vi "MouseMove.vi"(8 "Coords":T1, 9 "ActTool":i32, 10 "StartPoints":cluster{i16, i16}[](array[cluster]), 11 "reference":refnum<vi>) -> ()   [LabVIEW 2015, in "MyGraph.xctl"]
uses:
  MyGraph.xctl
  <vilib>/Utility/miscctls.llb/LVPoint32TypeDef.ctl
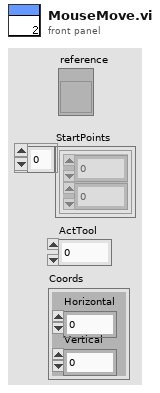
[diagram p1: front panel]
types:
  T1 = typedef "LVPoint32TypeDef.ctl" = cluster{"Horizontal":i32, "Vertical":i32}
  T2 = cluster{"left":i16, "top":i16, "right":i16, "bottom":i16}
  T3 = typedef "LVRectTypeDef.ctl" = cluster{"Left":i16, "Top":i16, "Right":i16, "Bottom":i16}
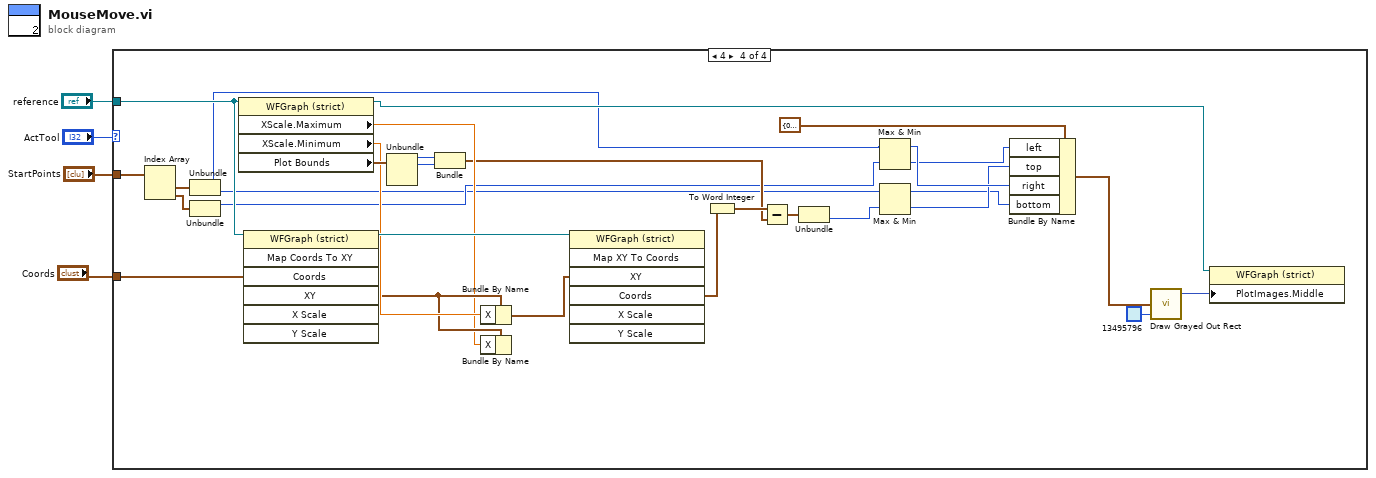
[diagram p0: block diagram]
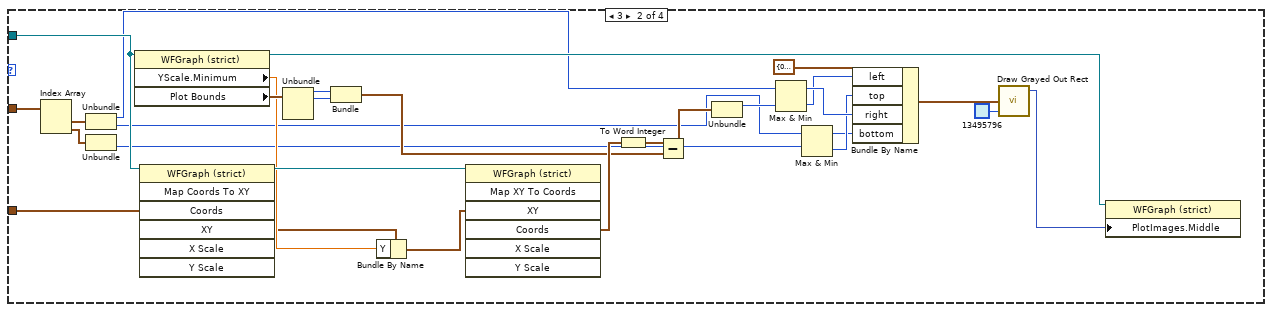
[diagram p3: hidden frame]
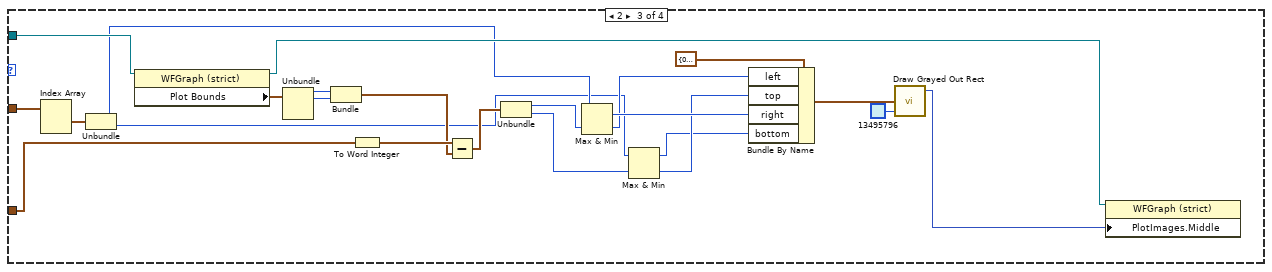
[diagram p4: hidden frame]
diagram:
  n1 = case shown="4" "ActTool" {
    tunnel: "StartPoints" -> [_ w16 w44 w67]
    tunnel: "reference" -> [_ w15 w43 w66]
    tunnel: "Coords" -> [_ w14 w42 w65]
    frame 0, Default {
    }
    frame 3 {
      n2 = Index Array(array=w16) -> (element #1=w22:cluster{i16, i16}, element #2=w21:cluster{i16, i16})  [unwired: 2 in]
      n3 = Unbundle(w22) -> (w12:i16, w7:i16)
      n4 = Unbundle(w21) -> (w8:i16)  [unwired: 1 out]
      n5 = property class="WFGraph (strict)"(reference=w15) -> (reference out=w18:refnum<vi>, "YScale.Minimum"=w28:dbl, "Plot Bounds"=w33:T3)  [unwired: 1 in, 1 out]
      n6 = invoke class="WFGraph (strict)" method="Map Coords To XY"(reference=w15, "Coords"=w14) -> (reference out=w29:refnum<vi>, "XY"=w27:cluster{"X":dbl, "Y":dbl})  [unwired: 5 in, 5 out]
      n7 = Unbundle(w33) -> ("Left"=w32:i16, "Top"=w31:i16)  [unwired: 2 out]
      n8 = Bundle("Left"=w32, "Top"=w31) -> (w24:cluster{"Left":i16, "Top":i16})  [unwired: 1 in]
      n9 = Bundle By Name(cluster=w27, "Y"=w28) -> (w26:cluster{"X":dbl, "Y":dbl})
      n10 = invoke class="WFGraph (strict)" method="Map XY To Coords"(reference=w29, "XY"=w26) -> ("Coords"=w25:T1)  [unwired: 5 in, 6 out]
      n11 = To Word Integer(number=w25) -> (16bit integer=w30:cluster{"Horizontal":i16, "Vertical":i16})
      n12 = Subtract(x=w30, y=w24) -> (x-y=w19:cluster{i16, i16})
      n13 = Unbundle(w19) -> (w11:i16)  [unwired: 1 out]
      n14 = Max & Min(x=w12, y=w11) -> (max(x,y)=w10:i16, min(x,y)=w9:i16)
      n15 = Max & Min(x=w7, y=w8) -> (max(x,y)=w5:i16, min(x,y)=w6:i16)
      n16 = Bundle By Name(cluster=T2 {"left"=0, "top"=0, "right"=0, "bottom"=0} ("rect"), "left"=w9, "top"=w6, "right"=w10, "bottom"=w5) -> (w20:T2)
      n17 = call <vilib>:"Draw Grayed Out Rect.vi"("color(black)"=u32 13495796, "rect"=w20) -> ("new picture"=w13:picture)  [unwired: 3 in]
      n18 = property class="WFGraph (strict)"(reference=w18, "PlotImages.Middle"=w13) -> ()  [unwired: 1 in, 2 out]
    }
    frame 2 {
      n19 = Index Array(array=w44) -> (element #1=w50:cluster{i16, i16})  [unwired: 2 in, 1 out]
      n20 = Unbundle(w50) -> (w40:i16, w36:i16)
      n21 = property class="WFGraph (strict)"(reference=w43) -> (reference out=w47:refnum<vi>, "Plot Bounds"=w56:T3)  [unwired: 1 in, 1 out]
      n22 = Unbundle(w56) -> ("Left"=w55:i16, "Top"=w54:i16)  [unwired: 2 out]
      n23 = Bundle("Left"=w55, "Top"=w54) -> (w52:cluster{"Left":i16, "Top":i16})  [unwired: 1 in]
      n24 = To Word Integer(number=w42) -> (16bit integer=w53:cluster{"Horizontal":i16, "Vertical":i16})
      n25 = Subtract(x=w53, y=w52) -> (x-y=w48:cluster{i16, i16})
      n26 = Unbundle(w48) -> (w41:i16, w37:i16)
      n27 = Max & Min(x=w40, y=w41) -> (max(x,y)=w39:i16, min(x,y)=w38:i16)
      n28 = Max & Min(x=w36, y=w37) -> (max(x,y)=w34:i16, min(x,y)=w35:i16)
      n29 = Bundle By Name(cluster=T2 {"left"=0, "top"=0, "right"=0, "bottom"=0} ("rect"), "left"=w38, "top"=w35, "right"=w39, "bottom"=w34) -> (w49:T2)
      n30 = call <vilib>:"Draw Grayed Out Rect.vi"("color(black)"=u32 13495796, "rect"=w49) -> ("new picture"=w45:picture)  [unwired: 3 in]
      n31 = property class="WFGraph (strict)"(reference=w47, "PlotImages.Middle"=w45) -> ()  [unwired: 1 in, 2 out]
    }
    frame 4 {
      n32 = Index Array(array=w67) -> (element #1=w74:cluster{i16, i16}, element #2=w73:cluster{i16, i16})  [unwired: 2 in]
      n33 = Unbundle(w74) -> (w64:i16, w60:i16)
      n34 = Unbundle(w73) -> (w63:i16)  [unwired: 1 out]
      n35 = property class="WFGraph (strict)"(reference=w66) -> (reference out=w70:refnum<vi>, "XScale.Maximum"=w79:dbl, "XScale.Minimum"=w81:dbl, "Plot Bounds"=w86:T3)  [unwired: 1 in, 1 out]
      n36 = invoke class="WFGraph (strict)" method="Map Coords To XY"(reference=w66, "Coords"=w65) -> (reference out=w82:refnum<vi>, "XY"=w80:cluster{"X":dbl, "Y":dbl})  [unwired: 5 in, 5 out]
      n37 = Unbundle(w86) -> ("Left"=w85:i16, "Top"=w84:i16)  [unwired: 2 out]
      n38 = Bundle("Left"=w85, "Top"=w84) -> (w76:cluster{"Left":i16, "Top":i16})  [unwired: 1 in]
      n39 = Bundle By Name(cluster=w80, "X"=w81) -> (w78:cluster{"X":dbl, "Y":dbl})
      n40 = Bundle By Name(cluster=w80, "X"=w79) -> ()  [unwired: 1 out]
      n41 = invoke class="WFGraph (strict)" method="Map XY To Coords"(reference=w82, "XY"=w78) -> ("Coords"=w77:T1)  [unwired: 5 in, 6 out]
      n42 = To Word Integer(number=w77) -> (16bit integer=w83:cluster{"Horizontal":i16, "Vertical":i16})
      n43 = Subtract(x=w83, y=w76) -> (x-y=w71:cluster{i16, i16})
      n44 = Unbundle(w71) -> (w59:i16)  [unwired: 1 out]
      n45 = Max & Min(x=w64, y=w63) -> (max(x,y)=w62:i16, min(x,y)=w61:i16)
      n46 = Max & Min(x=w60, y=w59) -> (max(x,y)=w57:i16, min(x,y)=w58:i16)
      n47 = Bundle By Name(cluster=T2 {"left"=0, "top"=0, "right"=0, "bottom"=0} ("rect"), "left"=w61, "top"=w58, "right"=w62, "bottom"=w57) -> (w72:T2)
      n48 = call <vilib>:"Draw Grayed Out Rect.vi"("color(black)"=u32 13495796, "rect"=w72) -> ("new picture"=w68:picture)  [unwired: 3 in]
      n49 = property class="WFGraph (strict)"(reference=w70, "PlotImages.Middle"=w68) -> ()  [unwired: 1 in, 2 out]
    }
  }
